vi "配方编辑.vi"() -> ()   [LabVIEW 2013]
uses:
  <vilib>/addons/database/Connection.llb/DB Tools Open Connec (String).vi
  <vilib>/addons/database/_DB Variant To Data/Database Variant To Data.xnode
  <vilib>/addons/database/NI_Database_API.lvlib
panel:
  in  "滚动步数":i32(c297)
  out "水平进度":u8(slide) min=1 max=5 scale=-1.0..5.0
  out "配方名称":string
  out "帮助状态":string
  in  "完成编辑":bool
  in  "设定步数":bool
  in  "插入步数":bool
  in  "删除步数":bool
  in  "删除功能":bool
  in  "编辑":bool
  in  "Function-Parameters":string[][](table)
  out "总步数":dbl
  out "当前步数":dbl
  in  "返回主界面":bool
  in  "Select-Fuctions":i32(listbox)
  in  "Available-Fuctions":i32(listbox)
  # "配 方 编 辑"
  # "of"
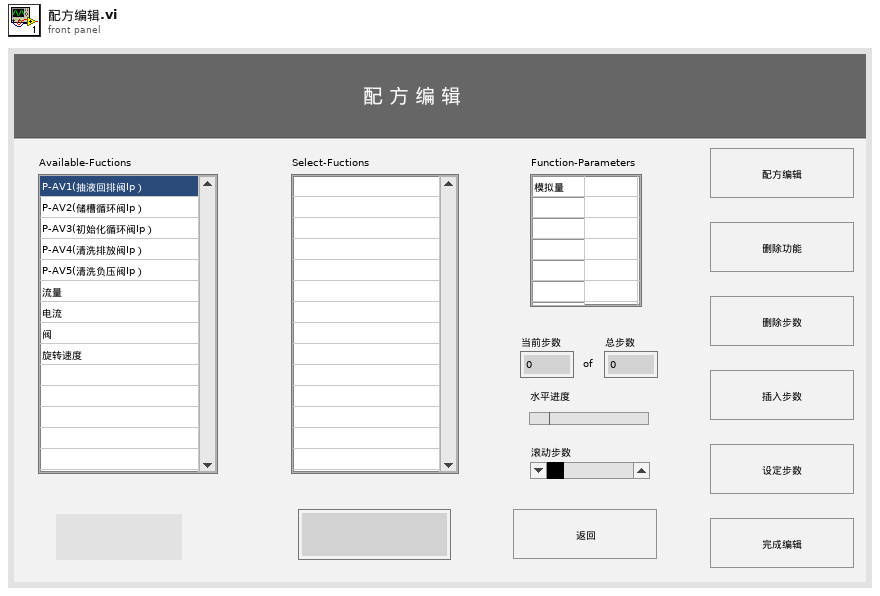
[diagram p1: front panel]
types:
  T1 = typedef "NI_Database_API.lvlib/Conn ObjectReference.ctl" = refnum<k1>
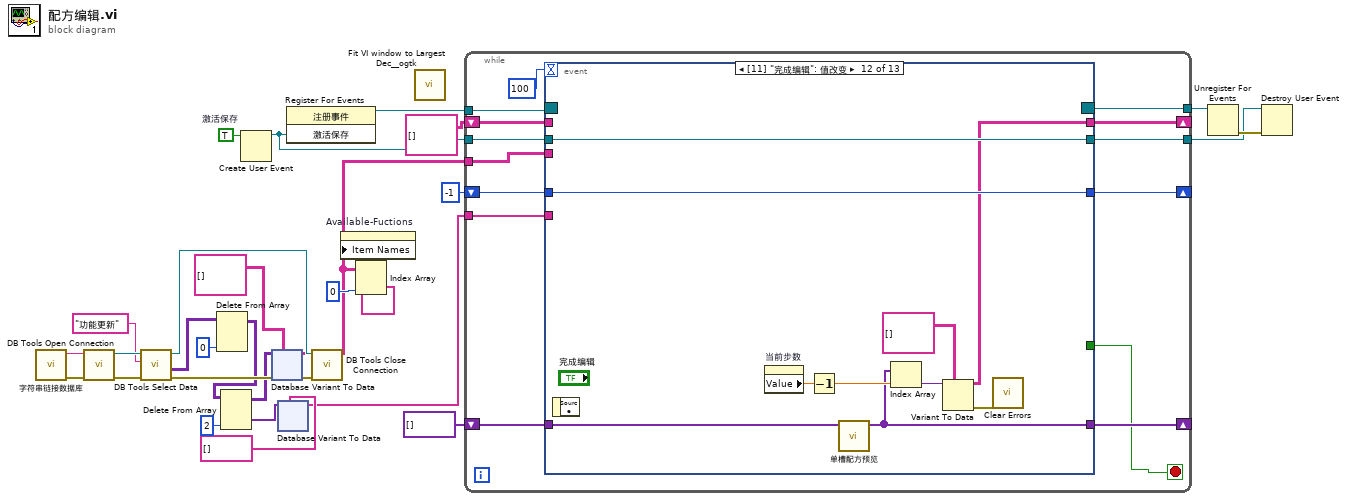
[diagram p0: block diagram]
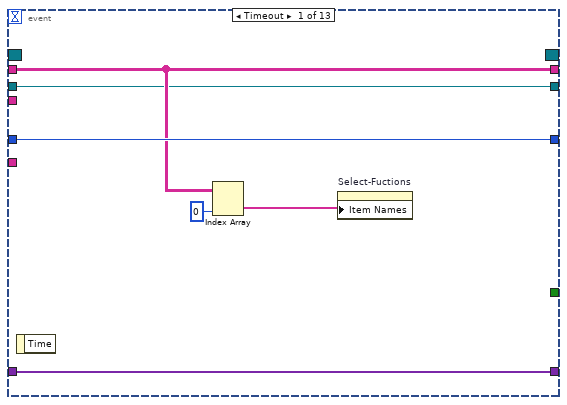
[diagram p2: hidden frame]
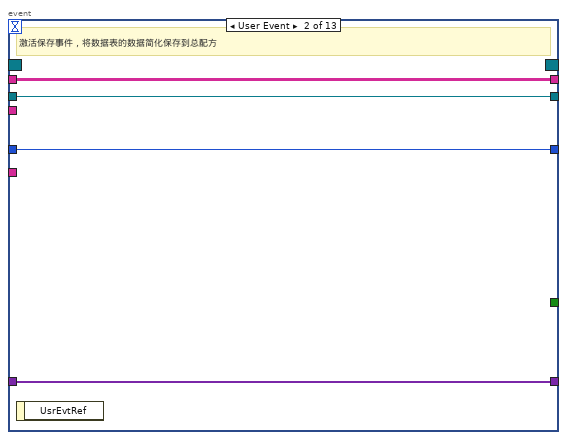
[diagram p3: hidden frame]
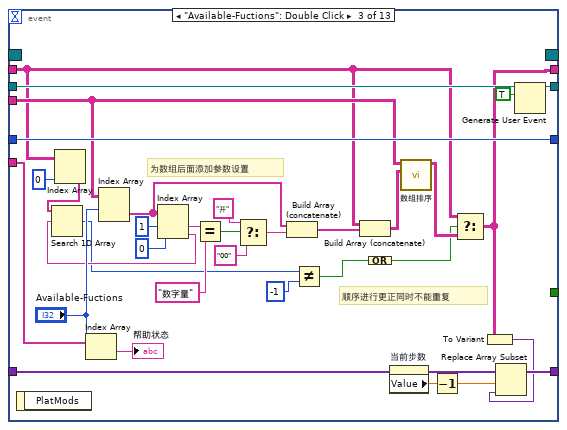
[diagram p4: hidden frame]
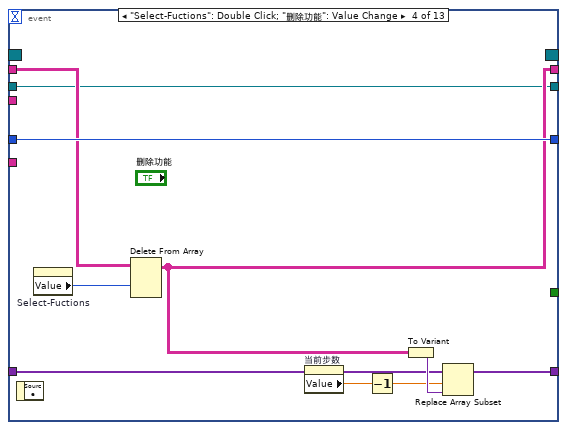
[diagram p5: hidden frame]
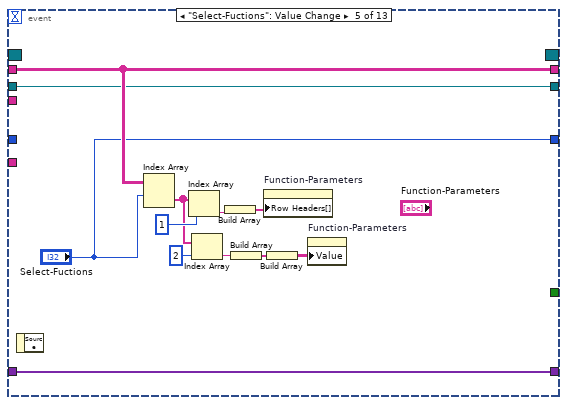
[diagram p6: hidden frame]
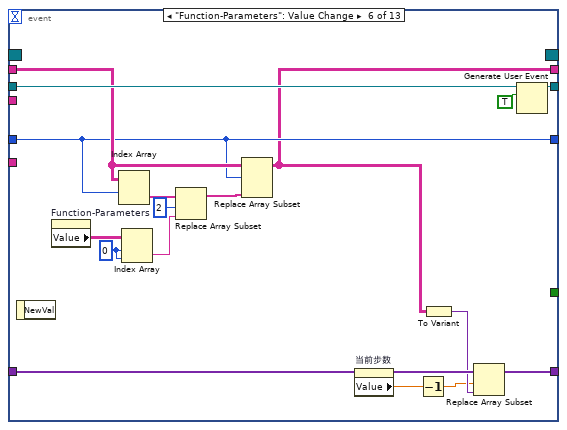
[diagram p7: hidden frame]
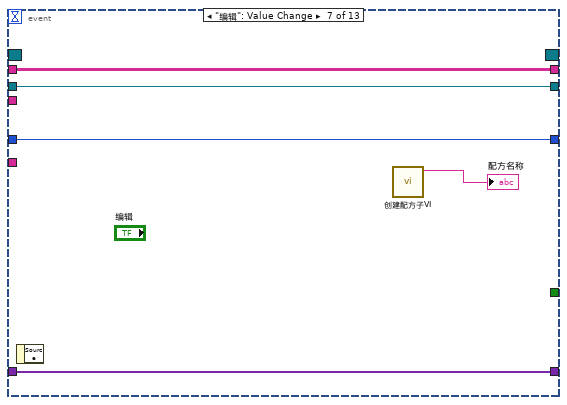
[diagram p8: hidden frame]
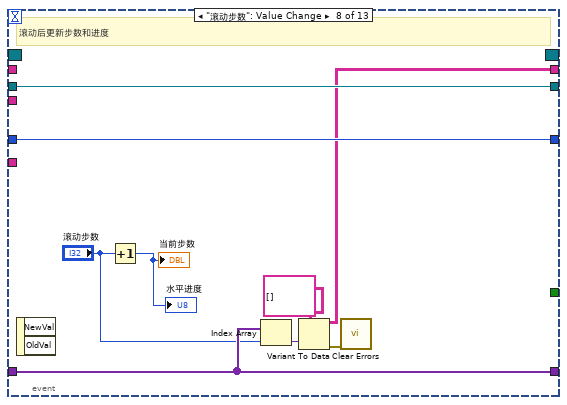
[diagram p9: hidden frame]
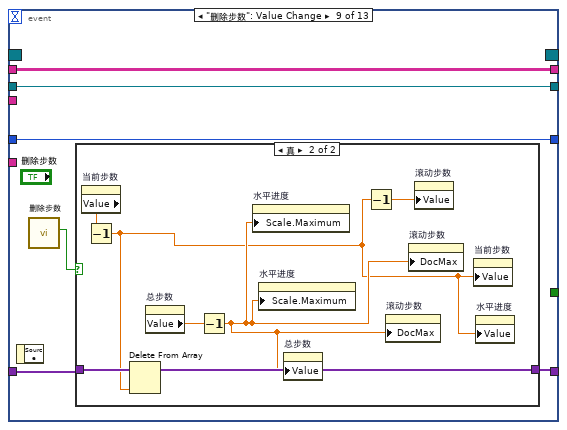
[diagram p10: hidden frame]
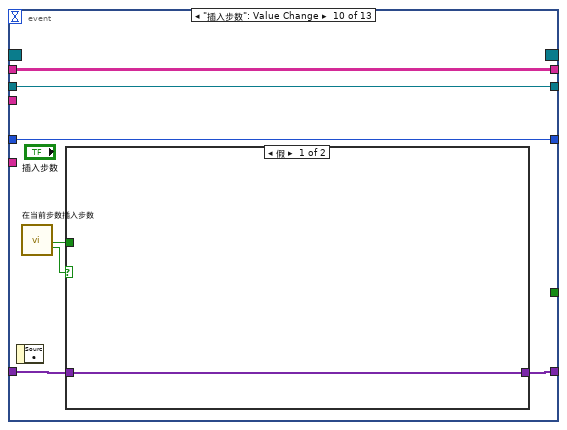
[diagram p12: hidden frame]
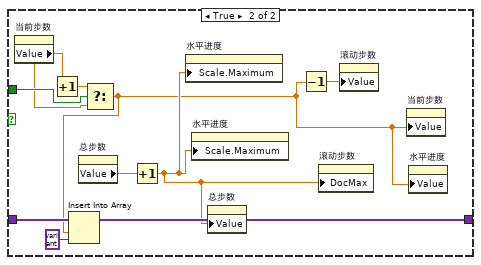
[diagram p13: hidden frame]
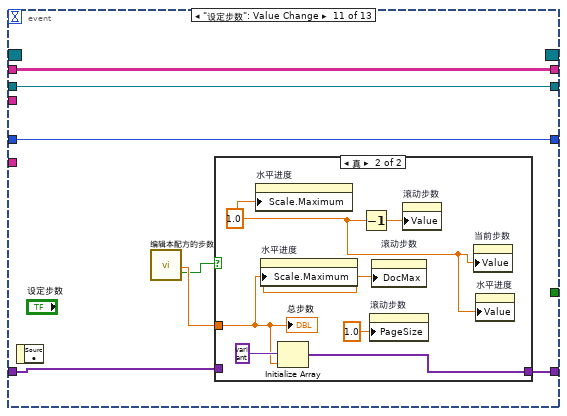
[diagram p14: hidden frame]
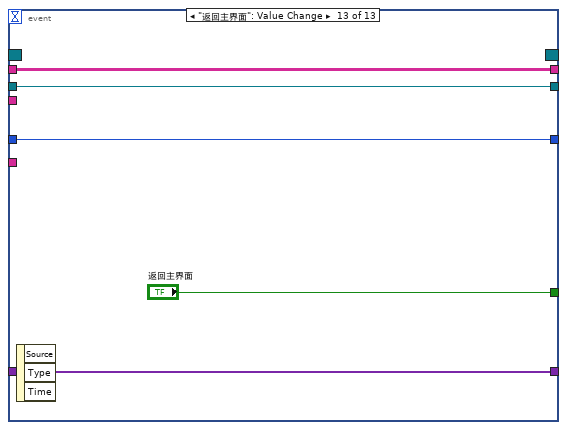
[diagram p16: hidden frame]
diagram:
  w6 = TRUE  # 激活保存
  n1 = call "字符串链接数据库.vi"() -> ("error out"=w28:errorcluster, "连接字符串"=w29:string)  [unwired: 10 in]
  n2 = call-poly <vilib>:"DB Tools Open Connection.vi"("error in (no error)"=w28, "connection information"=w29) -> ("error out"=w27:errorcluster, "connection reference"=w26:T1)  [unwired: 6 in]
  n3 = call <vilib>:"DB Tools Select Data.vi"("error in (no error)"=w27, "table"="功能更新", "connection reference"=w26) -> ("error out"=w24:errorcluster, "data"=w13:variant[][], "connection reference out"=w22:T1)  [unwired: 3 in]
  n4 = Delete From Array(array=w13, index (col)=0 ("禁用的索引 (列)")) -> (array with subset deleted=w12:variant[][])  [unwired: 2 in, 1 out]
  n5 = Delete From Array(array=w12, index (col)=2 ("禁用的索引 (列)")) -> (deleted portion=w8:variant[], array with subset deleted=w11:variant[][])  [unwired: 2 in]
  n6 = Create User Event(user event datatype=w6) -> (user event=w2:refnum<user-event>)  [unwired: 1 in, 1 out]
  n7 = xnode "Database Variant To Data"("database variant"=w11, "error in (no error)"=w24, "type"=string[][] []) -> ("data"=w18:string[][], "error out"=w23:errorcluster)
  n8 = xnode "Database Variant To Data"("database variant"=w8, "type"=string[] []) -> ("data"=w7:string[])  [unwired: 1 in, 1 out]
  n9 = register-events(w2) -> (reference out=w5:refnum<event-registration>)  [unwired: 2 in, 1 out]
  n10 = call <vilib>:"DB Tools Close Connection.vi"("error in (no error)"=w23, "connection reference"=w22) -> ()  [unwired: 5 in, 1 out]
  n11 = Index Array(array=w18, index (col)=0 ("禁用的索引 (列)")) -> (element=w19:string[])  [unwired: 1 in]
  n12 = property on="Available-Fuctions" class="LstBox (严格)"("Item Names"=w19) -> ()  [unwired: 2 in, 2 out]
  n13 = call <userlib>:"Fit VI window to Largest Dec__ogtk.vi"() -> ()  [unwired: 6 in, 2 out]
  n14 = while {
    tunnel: w18 -> [w43]
    shift-right: [w36] -> _
    shift-left: string[][] [] -> [w42]
    shift-right: [w40] -> _
    shift-left: -1 ("Available-Fuctions") -> [w39]
    shift-right: [w37] -> _
    shift-left: variant[] [] -> [w38]
    tunnel: w7 -> [w35]
    tunnel: w5 -> [w34]
    tunnel: [w33] -> w3
    tunnel: w2 -> [w32]
    tunnel: [w31] -> w1
    stop <- w30 stop-if-true
    n15 = event shown="[11] \"完成编辑\": 值改变" {
      selector: w34 -> [_ _ _ _ _ _ _ _ _ _ _ _ _]
      dyn-events: [_ _ _ _ _ _ _ _ _ _ _ _ _] -> w33
      timeout: 100 -> [_ _ _ _ _ _ _ _ _ _ _ _ _]
      tunnel: w43 -> [_ _ w66 _ _ _ _ _ _ _ _ _ _]
      tunnel: [w47 w53 w63 w95 w108 w112 w129 w131 w145 w159 w177 w187 w200] -> w36
      tunnel: w42 -> [w47 w53 w62 w90 w108 w115 w129 _ w145 w159 w177 _ w200]
      tunnel: [w49 w52 w87 w96 "Select-Fuctions" w114 w130 w139 w144 w160 w178 w195 w199] -> w40
      tunnel: w39 -> [w49 w52 w87 w96 _ w114 w130 w139 w144 w160 w178 w195 w199]
      tunnel: w38 -> [w48 w51 w86 w93 w109 w125 w127 w136 w143 w158 w173 w193 w198]
      tunnel: [w48 w51 w85 w92 w109 w124 w127 w136 w142 w156 w176 w190 w198] -> w37
      tunnel: w35 -> [_ _ w83 _ _ _ _ _ _ _ _ _ _]
      tunnel: w32 -> [w44 w50 w82 w89 w98 w122 w126 w137 w140 w154 w172 w194 w197]
      tunnel: [w44 w50 w68 w89 w98 w122 w126 w137 w140 w154 w172 w194 w197] -> w31
      tunnel: [_ _ _ _ _ _ _ _ _ _ _ _ "返回主界面"] -> w30
      event Timeout {
        n16 = event-data() -> ()  [unwired: 1 in, 1 out]
        n17 = Index Array(array=w47, index (col)=0 ("禁用的索引 (列)")) -> (element=w45:string[])  [unwired: 1 in]
        n18 = property on="Select-Fuctions" class="LstBox (严格)"("Item Names"=w45) -> ()  [unwired: 2 in, 2 out]
      }
      event User Event {
        # "激活保存事件，将数据表的数据简化保存到总配方"
        n19 = event-data() -> ()  [unwired: 1 in, 1 out]
      }
      event "Available-Fuctions": Double Click {
        # "顺序进行更正同时不能重复"
        # "为数组后面添加参数设置"
        n20 = event-data() -> ()  [unwired: 1 in, 1 out]
        n21 = Index Array(array=w62, index (col)=0 ("禁用的索引 (列)")) -> (element=w60:string[])  [unwired: 1 in]
        n22 = Index Array(array=w83, index="Available-Fuctions") -> (element=→"帮助状态":string)
        n23 = Index Array(array=w66, index (row)="Available-Fuctions") -> (element=w73:string[])  [unwired: 1 in]
        n24 = Index Array(array=w73, index #1=1 ("索引"), index #2=0 ("索引")) -> (element #1=w79:string, element #2=w58:string)
        n25 = Search 1D Array(1D array=w60, element=w58) -> (index of element=w57:i32)  [unwired: 1 in]
        n26 = Equal?(x=w79, y="数字量") -> (x = y?=w77:bool)
        n27 = Select(t="开", s=w77, f="00") -> (s? t:f=w74:string)
        n28 = Build Array (concatenate)(w73, w74) -> (w72:string[])
        n29 = Not Equal?(x=w57, y=-1) -> (x != y?=w55:bool)
        n30 = Build Array (concatenate)(w62, w72) -> (w67:string[][])
        n31 = Compound Arithmetic op=OR(w55) -> (w54:bool)
        n32 = property on="当前步数" class="DigNum (严格)"() -> ("Value"=w71:dbl)  [unwired: 2 in, 2 out]
        n33 = call "数组排序.vi"("需要排列数据"=w67, "总数据"=w66) -> ("完成后数据"=w64:string[][])  [unwired: 9 in]
        n34 = Decrement(x=w71) -> (x-1=w65:dbl)
        n35 = Select(t=w62, s=w54, f=w64) -> (s? t:f=w63:string[][])
        n36 = To Variant(anything=w63) -> (Variant=w70:variant)
        n37 = Replace Array Subset(array=w86, new element=w70, index=w65) -> (w85:variant[])
        n38 = Generate User Event(user event=w82, event data cluster=TRUE ("激活保存")) -> (user event out=w68:refnum<user-event>)  [unwired: 2 in, 1 out]
      }
      event "Select-Fuctions": Double Click; "删除功能": Value Change {
        n39 = event-data() -> ()  [unwired: 1 in, 1 out]
        n40 = property on="Select-Fuctions" class="LstBox (严格)"() -> ("Value"=w97:i32)  [unwired: 2 in, 2 out]
        n41 = Delete From Array(array=w90, index (row)=w97) -> (array with subset deleted=w95:string[][])  [unwired: 2 in, 1 out]
        n42 = property on="当前步数" class="DigNum (严格)"() -> ("Value"=w91:dbl)  [unwired: 2 in, 2 out]
        n43 = Decrement(x=w91) -> (x-1=w88:dbl)
        n44 = To Variant(anything=w95) -> (Variant=w94:variant)
        n45 = Replace Array Subset(array=w93, new element=w94, index=w88) -> (w92:variant[])
      }
      event "Select-Fuctions": Value Change {
        n46 = event-data() -> ()  [unwired: 1 in, 1 out]
        n47 = Index Array(array=w108, index (row)="Select-Fuctions") -> (element=w103:string[])  [unwired: 1 in]
        n48 = Index Array(array=w103, index=1 ("索引")) -> (element=w104:string)
        n49 = Index Array(array=w103, index=2 ("索引")) -> (element=w101:string)
        n50 = Build Array(w104) -> (w105:string[])
        n51 = Build Array(w101) -> (w100:string[])
        n52 = property on="Function-Parameters" class="Tbl (严格)"("Row Headers[]"=w105) -> ()  [unwired: 2 in, 2 out]
        n53 = Build Array(w100) -> (w99:string[][])
        n54 = property on="Function-Parameters" class="Tbl (严格)"("Value"=w99) -> ()  [unwired: 2 in, 2 out]
      }
      event "Function-Parameters": Value Change {
        w119 = 0 ("索引 (行)")
        n55 = event-data() -> ()  [unwired: 1 in, 1 out]
        n56 = property on="Function-Parameters" class="Tbl (严格)"() -> ("Value"=w120:string[][])  [unwired: 2 in, 2 out]
        n57 = Index Array(array=w115, index (row)=w114) -> (element=w118:string[])  [unwired: 1 in]
        n58 = Index Array(array=w120, index (row)=w119, index (col)=w119) -> (element=w116:string)
        n59 = Replace Array Subset(array=w118, new element=w116, index=2 ("索引")) -> (w113:string[])
        n60 = Replace Array Subset(array=w115, new element=w113, index (row)=w114) -> (w112:string[][])  [unwired: 1 in]
        n61 = property on="当前步数" class="DigNum (严格)"() -> ("Value"=w121:dbl)  [unwired: 2 in, 2 out]
        n62 = Decrement(x=w121) -> (x-1=w110:dbl)
        n63 = To Variant(anything=w112) -> (Variant=w111:variant)
        n64 = Replace Array Subset(array=w125, new element=w111, index=w110) -> (w124:variant[])
        n65 = Generate User Event(user event=w122, event data cluster=TRUE ("激活保存")) -> ()  [unwired: 2 in, 2 out]
      }
      event "编辑": Value Change {
        n66 = event-data() -> ()  [unwired: 1 in, 1 out]
        n67 = call "创建配方子VI.vi"() -> ("配方编号"=→"配方名称":string)  [unwired: 10 in]
      }
      event "滚动步数": Value Change {
        # "滚动后更新步数和进度"
        n68 = event-data() -> ()  [unwired: 1 in, 2 out]
        n69 = Increment(x="滚动步数") -> (x+1=→"当前步数" →"水平进度":i32)
        n70 = Index Array(array=w136, index="滚动步数") -> (element=w134:variant)
        n71 = Variant To Data(type=string[][] [], Variant=w134) -> (data=w131:string[][], error out=w132:errorcluster)  [unwired: 1 in]
        n72 = call <vilib>:"Clear Errors.vi"("error in (no error)"=w132) -> ()  [unwired: 6 in, 1 out]
      }
      event "删除步数": Value Change {
        n73 = event-data() -> ()  [unwired: 1 in, 1 out]
        n74 = call "删除步数"() -> ("确定"=w141:bool)  [unwired: 10 in, 1 out]
        n75 = case shown="真" w141 {
          tunnel: w143 -> [w146 w152]
          tunnel: [w146 w150] -> w142
          frame False {
          }
          frame True {
            n76 = property on="当前步数" class="DigNum (严格)"() -> ("Value"=w151:dbl)  [unwired: 2 in, 2 out]
            n77 = Decrement(x=w151) -> (x-1=w148:dbl)
            n78 = Delete From Array(array=w152, index=w148) -> (array with subset deleted=w150:variant[])  [unwired: 1 in, 1 out]
            n79 = property on="总步数" class="DigNum (严格)"() -> ("Value"=w153:dbl)  [unwired: 2 in, 2 out]
            n80 = Decrement(x=w153) -> (x-1=w149:dbl)
            n81 = property on="水平进度" class="Slide (严格)"("Scale.Maximum"=w149) -> ()  [unwired: 2 in, 2 out]
            n82 = property on="水平进度" class="Slide (严格)"("Scale.Maximum"=w149) -> ()  [unwired: 2 in, 2 out]
            n83 = property on="总步数" class="DigNum (严格)"("Value"=w149) -> ()  [unwired: 2 in, 2 out]
            n84 = Decrement(x=w148) -> (x-1=w147:dbl)
            n85 = property on="滚动步数" class="Scroll (严格)"("DocMax"=w149) -> ()  [unwired: 2 in, 2 out]
            n86 = property on="滚动步数" class="Scroll (严格)"("DocMax"=w149) -> ()  [unwired: 2 in, 2 out]
            n87 = property on="滚动步数" class="Scroll (严格)"("Value"=w147) -> ()  [unwired: 2 in, 2 out]
            n88 = property on="当前步数" class="DigNum (严格)"("Value"=w148) -> ()  [unwired: 2 in, 2 out]
            n89 = property on="水平进度" class="Slide (严格)"("Value"=w148) -> ()  [unwired: 2 in, 2 out]
          }
        }
      }
      event "插入步数": Value Change {
        n90 = event-data() -> ()  [unwired: 1 in, 1 out]
        n91 = call "在当前步数插入步数"() -> ("当前步数往前插入？"=w157:bool, "确定插入步数"=w155:bool)  [unwired: 17 in, 1 out]
        n92 = case shown="假" w155 {
          tunnel: w158 -> [w161 w171]
          tunnel: w157 -> [_ w170]
          tunnel: [w161 w168] -> w156
          frame False {
          }
          frame True {
            n93 = property on="当前步数" class="DigNum (严格)"() -> ("Value"=w165:dbl)  [unwired: 2 in, 2 out]
            n94 = Increment(x=w165) -> (x+1=w166:dbl)
            n95 = property on="总步数" class="DigNum (严格)"() -> ("Value"=w167:dbl)  [unwired: 2 in, 2 out]
            n96 = Select(t=w166, s=w170, f=w165) -> (s? t:f=w163:dbl)
            n97 = Insert Into Array(array=w171, index=w163, new element=variant ("新元素/子数组")) -> (w168:variant[])
            n98 = Increment(x=w167) -> (x+1=w164:dbl)
            n99 = property on="水平进度" class="Slide (严格)"("Scale.Maximum"=w164) -> ()  [unwired: 2 in, 2 out]
            n100 = property on="水平进度" class="Slide (严格)"("Scale.Maximum"=w164) -> ()  [unwired: 2 in, 2 out]
            n101 = property on="总步数" class="DigNum (严格)"("Value"=w164) -> ()  [unwired: 2 in, 2 out]
            n102 = Decrement(x=w163) -> (x-1=w162:dbl)
            n103 = property on="滚动步数" class="Scroll (严格)"("DocMax"=w164) -> ()  [unwired: 2 in, 2 out]
            n104 = property on="滚动步数" class="Scroll (严格)"("Value"=w162) -> ()  [unwired: 2 in, 2 out]
            n105 = property on="当前步数" class="DigNum (严格)"("Value"=w163) -> ()  [unwired: 2 in, 2 out]
            n106 = property on="水平进度" class="Slide (严格)"("Value"=w163) -> ()  [unwired: 2 in, 2 out]
          }
        }
      }
      event "设定步数": Value Change {
        n107 = event-data() -> ()  [unwired: 1 in, 1 out]
        n108 = call "编辑本配方的步数"() -> ("请输入步数"=w175:dbl, "确定"=w174:bool)  [unwired: 17 in, 1 out]
        n109 = case shown="真" w174 {
          tunnel: [w179 w183] -> w176
          tunnel: w175 -> [_ w182]
          tunnel: w173 -> [w179 _]
          frame False {
          }
          frame True {
            w181 = 1.0 ("数据输入界限:最小值")
            n110 = property on="水平进度" class="Slide (严格)"("Scale.Maximum"=w181) -> ()  [unwired: 2 in, 2 out]
            n111 = property on="水平进度" class="Slide (严格)"("Scale.Maximum"=w182) -> ()  [unwired: 2 in, 2 out]
            n112 = Initialize Array(variant ("变体"), w182) -> (w183:variant[])
            n113 = Decrement(x=w181) -> (x-1=w180:dbl)
            n114 = property on="滚动步数" class="Scroll (严格)"("PageSize"=1.0 ("页大小")) -> ()  [unwired: 2 in, 2 out]
            n115 = property on="滚动步数" class="Scroll (严格)"("DocMax"=w182) -> ()  [unwired: 2 in, 2 out]
            n116 = property on="滚动步数" class="Scroll (严格)"("Value"=w180) -> ()  [unwired: 2 in, 2 out]
            n117 = property on="当前步数" class="DigNum (严格)"("Value"=w181) -> ()  [unwired: 2 in, 2 out]
            n118 = property on="水平进度" class="Slide (严格)"("Value"=w181) -> ()  [unwired: 2 in, 2 out]
            "总步数" <- w182
          }
        }
      }
      event "完成编辑": Value Change {
        n119 = event-data() -> ()  [unwired: 1 in, 1 out]
        n120 = property on="当前步数" class="DigNum (严格)"() -> ("Value"=w192:dbl)  [unwired: 2 in, 2 out]
        n121 = Decrement(x=w192) -> (x-1=w191:dbl)
        n122 = call "单槽配方预览.vi"("数组"=w193) -> ("返回数据"=w190:variant[])  [unwired: 10 in]
        n123 = Index Array(array=w190, index=w191) -> (element=w189:variant)
        n124 = Variant To Data(type=string[][] [], Variant=w189) -> (data=w187:string[][], error out=w186:errorcluster)  [unwired: 1 in]
        n125 = call <vilib>:"Clear Errors.vi"("error in (no error)"=w186) -> ()  [unwired: 6 in, 1 out]
      }
      event "返回主界面": Value Change {
        n126 = event-data() -> ()  [unwired: 1 in, 3 out]
      }
    }
  }
  n127 = Unregister For Events(event registration refnum=w3) -> (error out=w4:errorcluster)  [unwired: 1 in]
  n128 = Destroy User Event(user event=w1, error in=w4) -> ()  [unwired: 1 out]
